vi "GetEventHardpointActuatorWarningField.vi"(10 "Event Data":string, 11 "Cluster in":refnum<vi>) -> (3 "Array":string[](array[string]))   [LabVIEW 2016]
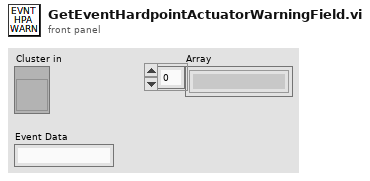
[diagram p1: front panel]
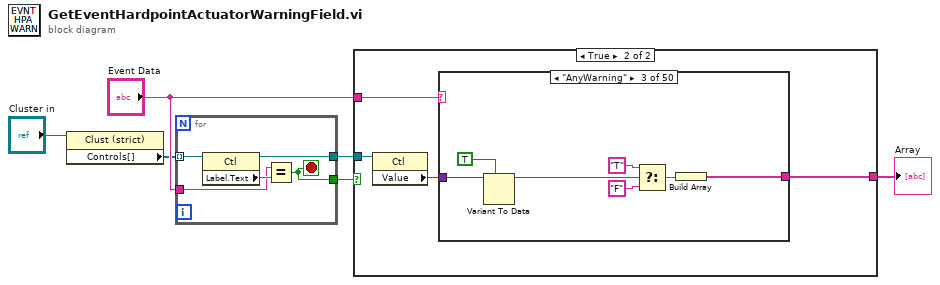
[diagram p0: block diagram]
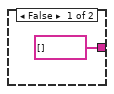
[diagram p2: hidden frame]
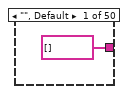
[diagram p3: hidden frame]
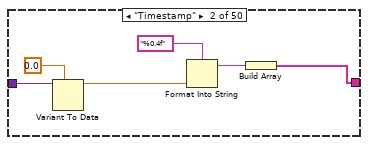
[diagram p4: hidden frame]
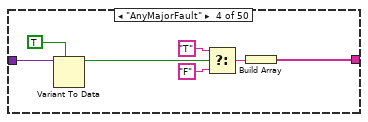
[diagram p5: hidden frame]
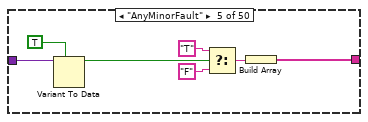
[diagram p6: hidden frame]
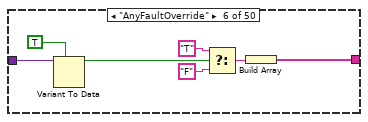
[diagram p7: hidden frame]
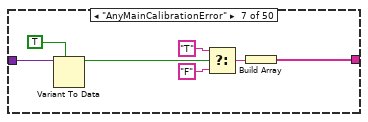
[diagram p8: hidden frame]
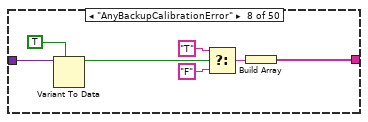
[diagram p9: hidden frame]
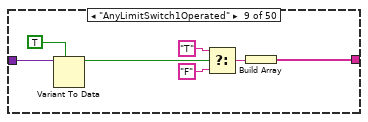
[diagram p10: hidden frame]
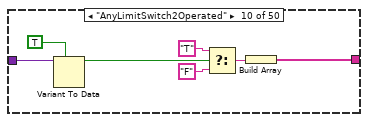
[diagram p11: hidden frame]
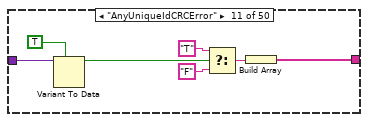
[diagram p12: hidden frame]
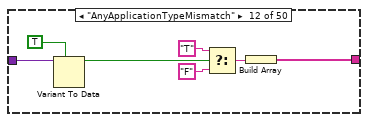
[diagram p13: hidden frame]
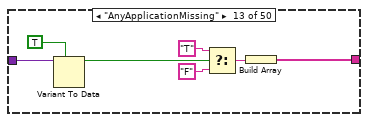
[diagram p14: hidden frame]
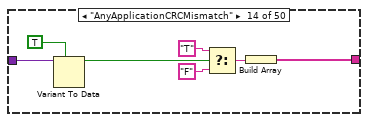
[diagram p15: hidden frame]
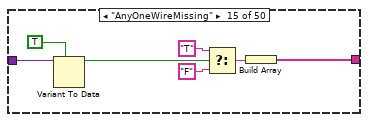
[diagram p16: hidden frame]
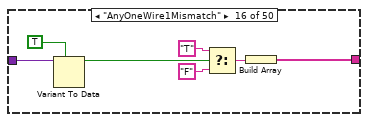
[diagram p17: hidden frame]
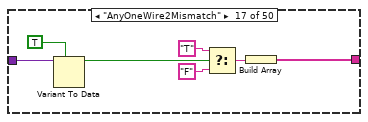
[diagram p18: hidden frame]
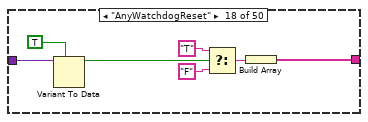
[diagram p19: hidden frame]
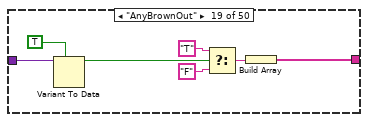
[diagram p20: hidden frame]
diagram:
  n1 = property on="Property Node" class="Clust (strict)"(reference="Cluster in") -> ("Controls[]"=w3:refnum<vi>[])  [unwired: 1 in, 2 out]
  n2 = for {
    tunnel: w3 -> [w11] mode=indexing
    tunnel: [w10] -> w5
    tunnel: "Event Data" -> [w8]
    tunnel: [w7] -> w6
    stop <- w7 stop-if-true
    n3 = property on="Property Node" class="Ctl"(reference=w11) -> (reference out=w10:refnum<vi>, "Label.Text"=w9:string)  [unwired: 1 in, 1 out]
    n4 = Equal?(x=w8, y=w9) -> (x = y?=w7:bool)
  }
  n5 = case shown="True" w6 {
    tunnel: "Event Data" -> [_ w16]
    tunnel: w5 -> [_ w15]
    tunnel: [string[] [] w13] -> w2
    frame False {
    }
    frame True {
      n6 = property on="Property Node" class="Ctl"(reference=w15) -> ("Value"=w14:variant)  [unwired: 1 in, 2 out]
      n7 = case shown="\"AnyWarning\"" w16 {
        tunnel: [string[] [] w21 w24 w31 w38 w45 w52 w59 w66 w73 w80 w87 w94 w101 w108 w115 w122 w129 w136 w143 w150 w157 w164 w171 w178 w185 w192 w200 w208 w216 w224 w232 w240 w248 w256 w264 w272 w280 w288 w296 w304 w312 w320 w328 w336 w344 w352 w360 w368 w379] -> w13
        tunnel: w14 -> [_ w19 w30 w37 w44 w51 w58 w65 w72 w79 w86 w93 w100 w107 w114 w121 w128 w135 w142 w149 w156 w163 w170 w177 w184 w191 w195 w203 w211 w219 w227 w235 w243 w251 w259 w267 w275 w283 w291 w299 w307 w315 w323 w331 w339 w347 w355 w363 w371 w377]
        frame "", Default {
        }
        frame "Timestamp" {
          n8 = Variant To Data(type=0.0, Variant=w19) -> (data=w20:dbl)  [unwired: 1 in, 1 out]
          n9 = Format Into String(format string="%0.4f", w20) -> (resulting string=w22:string)  [unwired: 2 in, 1 out]
          n10 = Build Array(w22) -> (w21:string[])
        }
        frame "AnyWarning" {
          n11 = Variant To Data(type=TRUE, Variant=w30) -> (data=w28:bool)  [unwired: 1 in, 1 out]
          n12 = Select(t="T", s=w28, f="F") -> (s? t:f=w25:string)
          n13 = Build Array(w25) -> (w24:string[])
        }
        frame "AnyMajorFault" {
          n14 = Variant To Data(type=TRUE, Variant=w37) -> (data=w35:bool)  [unwired: 1 in, 1 out]
          n15 = Select(t="T", s=w35, f="F") -> (s? t:f=w32:string)
          n16 = Build Array(w32) -> (w31:string[])
        }
        frame "AnyMinorFault" {
          n17 = Variant To Data(type=TRUE, Variant=w44) -> (data=w42:bool)  [unwired: 1 in, 1 out]
          n18 = Select(t="T", s=w42, f="F") -> (s? t:f=w39:string)
          n19 = Build Array(w39) -> (w38:string[])
        }
        frame "AnyFaultOverride" {
          n20 = Variant To Data(type=TRUE, Variant=w51) -> (data=w49:bool)  [unwired: 1 in, 1 out]
          n21 = Select(t="T", s=w49, f="F") -> (s? t:f=w46:string)
          n22 = Build Array(w46) -> (w45:string[])
        }
        frame "AnyMainCalibrationError" {
          n23 = Variant To Data(type=TRUE, Variant=w58) -> (data=w56:bool)  [unwired: 1 in, 1 out]
          n24 = Select(t="T", s=w56, f="F") -> (s? t:f=w53:string)
          n25 = Build Array(w53) -> (w52:string[])
        }
        frame "AnyBackupCalibrationError" {
          n26 = Variant To Data(type=TRUE, Variant=w65) -> (data=w63:bool)  [unwired: 1 in, 1 out]
          n27 = Select(t="T", s=w63, f="F") -> (s? t:f=w60:string)
          n28 = Build Array(w60) -> (w59:string[])
        }
        frame "AnyLimitSwitch1Operated" {
          n29 = Variant To Data(type=TRUE, Variant=w72) -> (data=w70:bool)  [unwired: 1 in, 1 out]
          n30 = Select(t="T", s=w70, f="F") -> (s? t:f=w67:string)
          n31 = Build Array(w67) -> (w66:string[])
        }
        frame "AnyLimitSwitch2Operated" {
          n32 = Variant To Data(type=TRUE, Variant=w79) -> (data=w77:bool)  [unwired: 1 in, 1 out]
          n33 = Select(t="T", s=w77, f="F") -> (s? t:f=w74:string)
          n34 = Build Array(w74) -> (w73:string[])
        }
        frame "AnyUniqueIdCRCError" {
          n35 = Variant To Data(type=TRUE, Variant=w86) -> (data=w84:bool)  [unwired: 1 in, 1 out]
          n36 = Select(t="T", s=w84, f="F") -> (s? t:f=w81:string)
          n37 = Build Array(w81) -> (w80:string[])
        }
        frame "AnyApplicationTypeMismatch" {
          n38 = Variant To Data(type=TRUE, Variant=w93) -> (data=w91:bool)  [unwired: 1 in, 1 out]
          n39 = Select(t="T", s=w91, f="F") -> (s? t:f=w88:string)
          n40 = Build Array(w88) -> (w87:string[])
        }
        frame "AnyApplicationMissing" {
          n41 = Variant To Data(type=TRUE, Variant=w100) -> (data=w98:bool)  [unwired: 1 in, 1 out]
          n42 = Select(t="T", s=w98, f="F") -> (s? t:f=w95:string)
          n43 = Build Array(w95) -> (w94:string[])
        }
        frame "AnyApplicationCRCMismatch" {
          n44 = Variant To Data(type=TRUE, Variant=w107) -> (data=w105:bool)  [unwired: 1 in, 1 out]
          n45 = Select(t="T", s=w105, f="F") -> (s? t:f=w102:string)
          n46 = Build Array(w102) -> (w101:string[])
        }
        frame "AnyOneWireMissing" {
          n47 = Variant To Data(type=TRUE, Variant=w114) -> (data=w112:bool)  [unwired: 1 in, 1 out]
          n48 = Select(t="T", s=w112, f="F") -> (s? t:f=w109:string)
          n49 = Build Array(w109) -> (w108:string[])
        }
        frame "AnyOneWire1Mismatch" {
          n50 = Variant To Data(type=TRUE, Variant=w121) -> (data=w119:bool)  [unwired: 1 in, 1 out]
          n51 = Select(t="T", s=w119, f="F") -> (s? t:f=w116:string)
          n52 = Build Array(w116) -> (w115:string[])
        }
        frame "AnyOneWire2Mismatch" {
          n53 = Variant To Data(type=TRUE, Variant=w128) -> (data=w126:bool)  [unwired: 1 in, 1 out]
          n54 = Select(t="T", s=w126, f="F") -> (s? t:f=w123:string)
          n55 = Build Array(w123) -> (w122:string[])
        }
        frame "AnyWatchdogReset" {
          n56 = Variant To Data(type=TRUE, Variant=w135) -> (data=w133:bool)  [unwired: 1 in, 1 out]
          n57 = Select(t="T", s=w133, f="F") -> (s? t:f=w130:string)
          n58 = Build Array(w130) -> (w129:string[])
        }
        frame "AnyBrownOut" {
          n59 = Variant To Data(type=TRUE, Variant=w142) -> (data=w140:bool)  [unwired: 1 in, 1 out]
          n60 = Select(t="T", s=w140, f="F") -> (s? t:f=w137:string)
          n61 = Build Array(w137) -> (w136:string[])
        }
        frame "AnyEventTrapReset" {
          n62 = Variant To Data(type=TRUE, Variant=w149) -> (data=w147:bool)  [unwired: 1 in, 1 out]
          n63 = Select(t="T", s=w147, f="F") -> (s? t:f=w144:string)
          n64 = Build Array(w144) -> (w143:string[])
        }
        frame "AnyMotorDriverFault" {
          n65 = Variant To Data(type=TRUE, Variant=w156) -> (data=w154:bool)  [unwired: 1 in, 1 out]
          n66 = Select(t="T", s=w154, f="F") -> (s? t:f=w151:string)
          n67 = Build Array(w151) -> (w150:string[])
        }
        frame "AnySSRPowerFault" {
          n68 = Variant To Data(type=TRUE, Variant=w163) -> (data=w161:bool)  [unwired: 1 in, 1 out]
          n69 = Select(t="T", s=w161, f="F") -> (s? t:f=w158:string)
          n70 = Build Array(w158) -> (w157:string[])
        }
        frame "AnyAuxPowerFault" {
          n71 = Variant To Data(type=TRUE, Variant=w170) -> (data=w168:bool)  [unwired: 1 in, 1 out]
          n72 = Select(t="T", s=w168, f="F") -> (s? t:f=w165:string)
          n73 = Build Array(w165) -> (w164:string[])
        }
        frame "AnySMCPowerFault" {
          n74 = Variant To Data(type=TRUE, Variant=w177) -> (data=w175:bool)  [unwired: 1 in, 1 out]
          n75 = Select(t="T", s=w175, f="F") -> (s? t:f=w172:string)
          n76 = Build Array(w172) -> (w171:string[])
        }
        frame "AnyILCFault" {
          n77 = Variant To Data(type=TRUE, Variant=w184) -> (data=w182:bool)  [unwired: 1 in, 1 out]
          n78 = Select(t="T", s=w182, f="F") -> (s? t:f=w179:string)
          n79 = Build Array(w179) -> (w178:string[])
        }
        frame "AnyBroadcastCounterWarning" {
          n80 = Variant To Data(type=TRUE, Variant=w191) -> (data=w189:bool)  [unwired: 1 in, 1 out]
          n81 = Select(t="T", s=w189, f="F") -> (s? t:f=w186:string)
          n82 = Build Array(w186) -> (w185:string[])
        }
        frame "MajorFault[6]" {
          n83 = Variant To Data(type=bool[] [], Variant=w195) -> (data=w193:bool[])  [unwired: 1 in, 1 out]
          n84 = for {
            tunnel: w193 -> [w199] mode=indexing
            tunnel: [w196] -> w192 mode=indexing
            n85 = Select(t="T", s=w199, f="F") -> (s? t:f=w196:string)
          }
        }
        frame "MinorFault[6]" {
          n86 = Variant To Data(type=bool[] [], Variant=w203) -> (data=w201:bool[])  [unwired: 1 in, 1 out]
          n87 = for {
            tunnel: w201 -> [w207] mode=indexing
            tunnel: [w204] -> w200 mode=indexing
            n88 = Select(t="T", s=w207, f="F") -> (s? t:f=w204:string)
          }
        }
        frame "FaultOverride[6]" {
          n89 = Variant To Data(type=bool[] [], Variant=w211) -> (data=w209:bool[])  [unwired: 1 in, 1 out]
          n90 = for {
            tunnel: w209 -> [w215] mode=indexing
            tunnel: [w212] -> w208 mode=indexing
            n91 = Select(t="T", s=w215, f="F") -> (s? t:f=w212:string)
          }
        }
        frame "MainCalibrationError[6]" {
          n92 = Variant To Data(type=bool[] [], Variant=w219) -> (data=w217:bool[])  [unwired: 1 in, 1 out]
          n93 = for {
            tunnel: w217 -> [w223] mode=indexing
            tunnel: [w220] -> w216 mode=indexing
            n94 = Select(t="T", s=w223, f="F") -> (s? t:f=w220:string)
          }
        }
        frame "BackupCalibrationError[6]" {
          n95 = Variant To Data(type=bool[] [], Variant=w227) -> (data=w225:bool[])  [unwired: 1 in, 1 out]
          n96 = for {
            tunnel: w225 -> [w231] mode=indexing
            tunnel: [w228] -> w224 mode=indexing
            n97 = Select(t="T", s=w231, f="F") -> (s? t:f=w228:string)
          }
        }
        frame "LimitSwitch1Operated[6]" {
          n98 = Variant To Data(type=bool[] [], Variant=w235) -> (data=w233:bool[])  [unwired: 1 in, 1 out]
          n99 = for {
            tunnel: w233 -> [w239] mode=indexing
            tunnel: [w236] -> w232 mode=indexing
            n100 = Select(t="T", s=w239, f="F") -> (s? t:f=w236:string)
          }
        }
        frame "LimitSwitch2Operated[6]" {
          n101 = Variant To Data(type=bool[] [], Variant=w243) -> (data=w241:bool[])  [unwired: 1 in, 1 out]
          n102 = for {
            tunnel: w241 -> [w247] mode=indexing
            tunnel: [w244] -> w240 mode=indexing
            n103 = Select(t="T", s=w247, f="F") -> (s? t:f=w244:string)
          }
        }
        frame "UniqueIdCRCError[6]" {
          n104 = Variant To Data(type=bool[] [], Variant=w251) -> (data=w249:bool[])  [unwired: 1 in, 1 out]
          n105 = for {
            tunnel: w249 -> [w255] mode=indexing
            tunnel: [w252] -> w248 mode=indexing
            n106 = Select(t="T", s=w255, f="F") -> (s? t:f=w252:string)
          }
        }
        frame "ApplicationTypeMismatch[6]" {
          n107 = Variant To Data(type=bool[] [], Variant=w259) -> (data=w257:bool[])  [unwired: 1 in, 1 out]
          n108 = for {
            tunnel: w257 -> [w263] mode=indexing
            tunnel: [w260] -> w256 mode=indexing
            n109 = Select(t="T", s=w263, f="F") -> (s? t:f=w260:string)
          }
        }
        frame "ApplicationMissing[6]" {
          n110 = Variant To Data(type=bool[] [], Variant=w267) -> (data=w265:bool[])  [unwired: 1 in, 1 out]
          n111 = for {
            tunnel: w265 -> [w271] mode=indexing
            tunnel: [w268] -> w264 mode=indexing
            n112 = Select(t="T", s=w271, f="F") -> (s? t:f=w268:string)
          }
        }
        frame "ApplicationCRCMismatch[6]" {
          n113 = Variant To Data(type=bool[] [], Variant=w275) -> (data=w273:bool[])  [unwired: 1 in, 1 out]
          n114 = for {
            tunnel: w273 -> [w279] mode=indexing
            tunnel: [w276] -> w272 mode=indexing
            n115 = Select(t="T", s=w279, f="F") -> (s? t:f=w276:string)
          }
        }
        frame "OneWireMissing[6]" {
          n116 = Variant To Data(type=bool[] [], Variant=w283) -> (data=w281:bool[])  [unwired: 1 in, 1 out]
          n117 = for {
            tunnel: w281 -> [w287] mode=indexing
            tunnel: [w284] -> w280 mode=indexing
            n118 = Select(t="T", s=w287, f="F") -> (s? t:f=w284:string)
          }
        }
        frame "OneWire1Mismatch[6]" {
          n119 = Variant To Data(type=bool[] [], Variant=w291) -> (data=w289:bool[])  [unwired: 1 in, 1 out]
          n120 = for {
            tunnel: w289 -> [w295] mode=indexing
            tunnel: [w292] -> w288 mode=indexing
            n121 = Select(t="T", s=w295, f="F") -> (s? t:f=w292:string)
          }
        }
        frame "OneWire2Mismatch[6]" {
          n122 = Variant To Data(type=bool[] [], Variant=w299) -> (data=w297:bool[])  [unwired: 1 in, 1 out]
          n123 = for {
            tunnel: w297 -> [w303] mode=indexing
            tunnel: [w300] -> w296 mode=indexing
            n124 = Select(t="T", s=w303, f="F") -> (s? t:f=w300:string)
          }
        }
        frame "WatchdogReset[6]" {
          n125 = Variant To Data(type=bool[] [], Variant=w307) -> (data=w305:bool[])  [unwired: 1 in, 1 out]
          n126 = for {
            tunnel: w305 -> [w311] mode=indexing
            tunnel: [w308] -> w304 mode=indexing
            n127 = Select(t="T", s=w311, f="F") -> (s? t:f=w308:string)
          }
        }
        frame "BrownOut[6]" {
          n128 = Variant To Data(type=bool[] [], Variant=w315) -> (data=w313:bool[])  [unwired: 1 in, 1 out]
          n129 = for {
            tunnel: w313 -> [w319] mode=indexing
            tunnel: [w316] -> w312 mode=indexing
            n130 = Select(t="T", s=w319, f="F") -> (s? t:f=w316:string)
          }
        }
        frame "EventTrapReset[6]" {
          n131 = Variant To Data(type=bool[] [], Variant=w323) -> (data=w321:bool[])  [unwired: 1 in, 1 out]
          n132 = for {
            tunnel: w321 -> [w327] mode=indexing
            tunnel: [w324] -> w320 mode=indexing
            n133 = Select(t="T", s=w327, f="F") -> (s? t:f=w324:string)
          }
        }
        frame "MotorDriverFault[6]" {
          n134 = Variant To Data(type=bool[] [], Variant=w331) -> (data=w329:bool[])  [unwired: 1 in, 1 out]
          n135 = for {
            tunnel: w329 -> [w335] mode=indexing
            tunnel: [w332] -> w328 mode=indexing
            n136 = Select(t="T", s=w335, f="F") -> (s? t:f=w332:string)
          }
        }
        frame "SSRPowerFault[6]" {
          n137 = Variant To Data(type=bool[] [], Variant=w339) -> (data=w337:bool[])  [unwired: 1 in, 1 out]
          n138 = for {
            tunnel: w337 -> [w343] mode=indexing
            tunnel: [w340] -> w336 mode=indexing
            n139 = Select(t="T", s=w343, f="F") -> (s? t:f=w340:string)
          }
        }
        frame "AuxPowerFault[6]" {
          n140 = Variant To Data(type=bool[] [], Variant=w347) -> (data=w345:bool[])  [unwired: 1 in, 1 out]
          n141 = for {
            tunnel: w345 -> [w351] mode=indexing
            tunnel: [w348] -> w344 mode=indexing
            n142 = Select(t="T", s=w351, f="F") -> (s? t:f=w348:string)
          }
        }
        frame "SMCPowerFault[6]" {
          n143 = Variant To Data(type=bool[] [], Variant=w355) -> (data=w353:bool[])  [unwired: 1 in, 1 out]
          n144 = for {
            tunnel: w353 -> [w359] mode=indexing
            tunnel: [w356] -> w352 mode=indexing
            n145 = Select(t="T", s=w359, f="F") -> (s? t:f=w356:string)
          }
        }
        frame "ILCFault[6]" {
          n146 = Variant To Data(type=bool[] [], Variant=w363) -> (data=w361:bool[])  [unwired: 1 in, 1 out]
          n147 = for {
            tunnel: w361 -> [w367] mode=indexing
            tunnel: [w364] -> w360 mode=indexing
            n148 = Select(t="T", s=w367, f="F") -> (s? t:f=w364:string)
          }
        }
        frame "BroadcastCounterWarning[6]" {
          n149 = Variant To Data(type=bool[] [], Variant=w371) -> (data=w369:bool[])  [unwired: 1 in, 1 out]
          n150 = for {
            tunnel: w369 -> [w375] mode=indexing
            tunnel: [w372] -> w368 mode=indexing
            n151 = Select(t="T", s=w375, f="F") -> (s? t:f=w372:string)
          }
        }
        frame "priority" {
          n152 = Variant To Data(type=0, Variant=w377) -> (data=w378:i32)  [unwired: 1 in, 1 out]
          n153 = Format Into String(format string="%d", w378) -> (resulting string=w380:string)  [unwired: 2 in, 1 out]
          n154 = Build Array(w380) -> (w379:string[])
        }
      }
    }
  }
  "Array" <- w2
